vi "Initialize.vi"(8 "error in (no error)":errorcluster, 11 "UDPlog Transfer Tx User Interface in":refnum<class "UDPlog Transfer Tx User Interface.lvclass">) -> (0 "error out":errorcluster, 3 "UDPlog Transfer Tx User Interface out":refnum<class "UDPlog Transfer Tx User Interface.lvclass">)   [LabVIEW 2023, in "UDPlog.lvlib" / "UDPlog Transfer Tx User Interface.lvclass"]
uses:
  UDPlog Transfer Tx User Interface.lvclass
  C:/Users/Public/Documents/National Instruments/NI VeriStand 2023/Custom Devices/Data Sharing Framework/Linux_x64/DSF Core.lvlibp/Classes/User Interface/User Interface.lvclass
  Configurations/Tx Transfer/UDPlog Transfer Tx Configuration.lvclass
  C:/Users/Public/Documents/National Instruments/NI VeriStand 2023/Custom Devices/Data Sharing Framework/Linux_x64/DSF Core.lvlibp/Classes/Configuration/Configuration.lvclass
  Users/Public/Documents/National Instruments/NI VeriStand 2023/Custom Devices/Data Sharing Framework/Linux_x64/DSF Core.lvlibp/Classes/User Interface/User Interface.lvclass
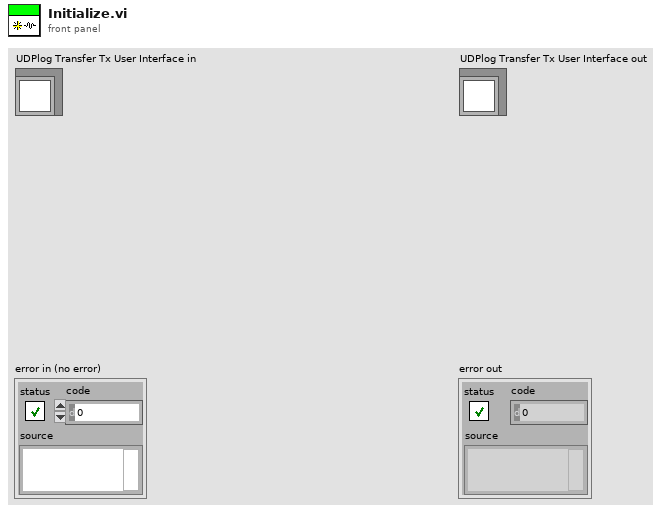
[diagram p1: front panel]
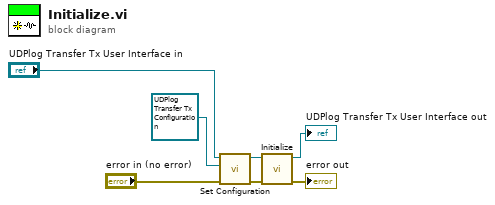
[diagram p0: block diagram]
diagram:
  n1 = call "Set Configuration.vi"("error in (no error)"="error in (no error)", "configuration"=refnum<class "UDPlog Transfer Tx Configuration.lvclass"> refnum ("UDPlog.lvlib:UDPlog Transfer Tx Configuration.lvclass"), "User Interface in"="UDPlog Transfer Tx User Interface in") -> ("error out"=w3:errorcluster, "User Interface out"=w4:refnum<class "UDPlog Transfer Tx User Interface.lvclass">)  [unwired: 7 in]
  n2 = call-parent "Initialize.vi"("error in (no error)"=w3, "User Interface in"=w4) -> ("error out"=→"error out":errorcluster, "User Interface out"=→"UDPlog Transfer Tx User Interface out":refnum<class "UDPlog Transfer Tx User Interface.lvclass">)  [unwired: 8 in]
